vi "Test Open Close.vi"() -> ()   [LabVIEW 2019, in "instrument.PPMS.lvclass"]
uses:
  instrument.PPMS.lvclass
  Typedefs/Select PPMS--Enum.ctl
  Typedefs/PPMS.getAll--cluster.ctl
panel:
  out "current time":timestamp=timestamp(3822909350.3365417 s since 1904-01-01)
  out "Numeric":i32=27
  out "Paths":string="llab_039:v004(PPMSim--Chamber Status())\nllab_039:d005(PPMSim--Helium Level(%))\nllab_039:d007(PPMSim--Temperature(K))\nllab_039:v002(PPMSim--Temperature Status())\nllab_039:d006(PPMSim--Magnetic Field(T))\nllab_039:v003(PPMSim--Magnet Status())"
  out "output cluster":variant=variant(cluster{"Chamber Status":string, "Helium Level":dbl, "Temperature":dbl, "Temperature Status":string, "Magnetic Field":dbl, "Magnet Status":string} {"Chamber Status"="ChamberUnknown", "Helium Level"=0.0, "Temperature"=0.0, "Temperature Status"="TemperatureUnknown", "Magnetic Field"=0.0, "Magnet Status"="MagnetUnknown"})
  out "getAll":T1={"Chamber Status"="ChamberUnknown", "Helium Level"=0.0, "Temperature"=0.0, "Temperature Status"="TemperatureUnknown", "Magnetic Field"=0.0, "Magnet Status"="MagnetUnknown", "Position"=0.0}
  in  "stop":bool
  in  "Select PPMS":T2=enum."Simulate OptiCool"
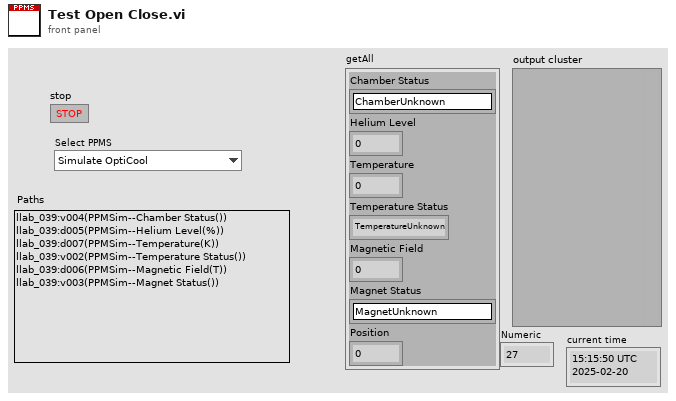
[diagram p1: front panel]
types:
  T1 = typedef "instrument.PPMS.lvclass/PPMS.getAll--cluster.ctl" = cluster{"Chamber Status":string, "Helium Level":dbl, "Temperature":dbl, "Temperature Status":string, "Magnetic Field":dbl, "Magnet Status":string, "Position":dbl}
  T2 = typedef "instrument.PPMS.lvclass/Select PPMS--Enum.ctl" = enum16{"PPMS1", "PPMS2", "PPMS3", "OptiCool", "Simulate PPMS", "Simulate OptiCool"}
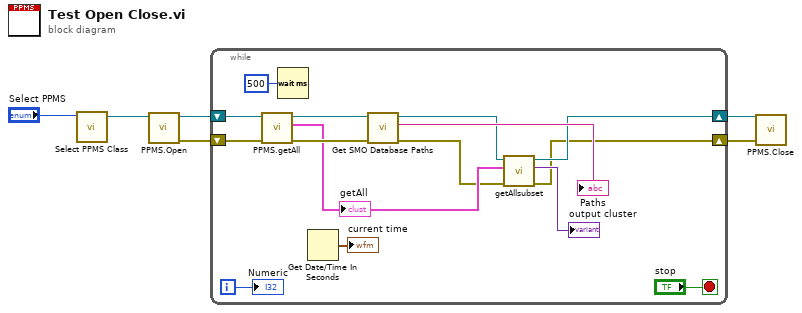
[diagram p0: block diagram]
diagram:
  n1 = call "Select PPMS Class.vi"("Select PPMS"="Select PPMS") -> ("instrument.PPMS out"=w6:refnum<class "instrument.PPMS.lvclass">)  [unwired: 9 in, 1 out]
  n2 = call "PPMS.Open.vi"("instrument.PPMS in"=w6) -> ("error out"=w3:errorcluster, "instrument.PPMS out"=w4:refnum<class "instrument.PPMS.lvclass">)  [unwired: 9 in]
  n3 = while {
    shift-right: [w12] -> w2
    shift-left: w4 -> [w19]
    shift-right: [w9] -> w1
    shift-left: w3 -> [w18]
    i -> [w8]
    stop <- "stop" stop-if-true
    n4 = call-dynamic "PPMS.getAll.vi"("error in (no error)"=w18, "instrument.PPMS in"=w19) -> ("error out"=w15:errorcluster, "getAll"=w13:T1, "instrument.PPMS out"=w14:refnum<class "instrument.PPMS.lvclass">)  [unwired: 7 in]
    "getAll" <- w13
    n5 = Wait (ms)(milliseconds to wait=u32 500) -> ()  [unwired: 1 out]
    n6 = Get Date/Time In Seconds() -> (seconds since 1Jan1904=→"current time":timestamp)
    n7 = call-dynamic "Get SMO Database Paths.vi"("error in (no error)"=w15, "instrument.PPMS in"=w14) -> ("error out"=w10:errorcluster, "Paths"=→"Paths":string, "instrument.PPMS out"=w16:refnum<class "instrument.PPMS.lvclass">)  [unwired: 7 in]
    n8 = call-dynamic "getAllsubset.vi"("error in (no error)"=w10, "getAll"=w13, "instrument.PPMS in"=w16) -> ("error out"=w9:errorcluster, "output cluster"=→"output cluster":variant, "instrument.PPMS out"=w12:refnum<class "instrument.PPMS.lvclass">)  [unwired: 6 in]
    "Numeric" <- w8
  }
  n9 = call "PPMS.Close.vi"("error in (no error)"=w1, "instrument.PPMS in"=w2) -> ()  [unwired: 8 in, 2 out]
